vi "Measure Trigger.vi"(0 "Intrument Handle[]":refnum<k15>[](array[refnum]), 5 "Channel Name":string[](array[string]), 11 "error in (no error)":errorcluster) -> (15 "error out":errorcluster)   [LabVIEW 2024, in "devicePowerSequencerCoreLogic.lvlib"]
doc: "Configure Measure Trigger"
uses:
  devicePowerSequencerCoreLogic.lvlib
  <instrlib>/niDCPower/nidcpower.llb/niDCPower Configure Digital Edge Measure Trigger With Channels.vi
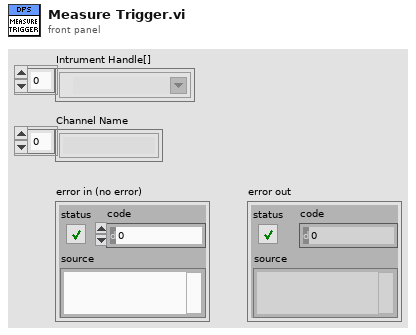
[diagram p1: front panel]
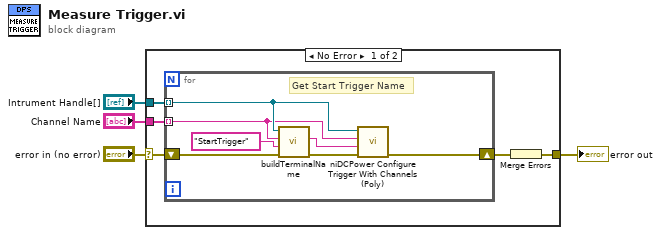
[diagram p0: block diagram]
diagram:
  n1 = case shown="No Error" "error in (no error)" {
    selector: "error in (no error)" -> [w5 w17]
    tunnel: "Intrument Handle[]" -> [w7 _]
    tunnel: [w8 w17] -> w2
    tunnel: "Channel Name" -> [w6 _]
    frame No Error {
      n2 = for {
        tunnel: w7 -> [w15] mode=indexing
        tunnel: w6 -> [w13] mode=indexing
        shift-right: [w16] -> w9
        shift-left: w5 -> [w12]
        # "Get Start Trigger Name"
        n3 = call "buildTerminalName.vi"("error in (no error)"=w12, "Local Terminal Name"="StartTrigger", "Channel Name"=w13, "session handle"=w15) -> ("error IO"=w11:errorcluster, "Fully Qualified Terminal Name"=w10:string)  [unwired: 5 in, 1 out]
        n4 = call-poly <instrlib>:"niDCPower Configure Trigger With Channels (Poly).vi"("error in (no error)"=w11, "input terminal"=w10, "channel name"=w13, "instrument handle"=w15) -> ("error out"=w16:errorcluster)  [unwired: 6 in, 1 out]
      }
      n5 = Merge Errors(w9) -> (w8:errorcluster)
    }
    frame Error {
    }
  }
  "error out" <- w2
